vi "UpdatePrefKnown.vi"(0 "PrefItemNode in":refnum<k20>, 1 "UpdateResult":T1, 2 "error in (no error)":errorcluster) -> (3 "PrefItemNode out":refnum<k20>, 4 "Updated XML":string, 5 "Not Current":bool, 6 "error out":errorcluster)   [LabVIEW 2013, in "SetListPrefs.lvclass"]
uses:
  SetListPrefs.lvclass
  <resource>/objmgr/DOMUserDefRef.rc
  UpdateResult.ctl
  <vilib>/regexp/Match Regular Expression.xnode
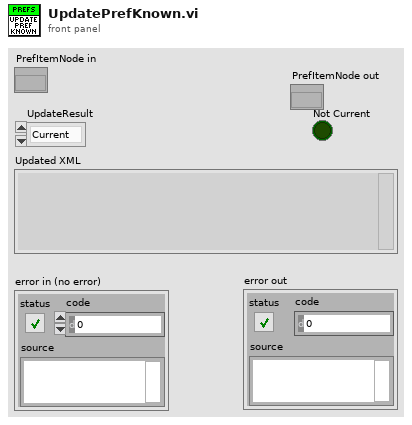
[diagram p1: front panel]
types:
  T1 = typedef "SetListPrefs.lvclass/UpdateResult.ctl" = enum16{"Current", "Old", "Unknown"}
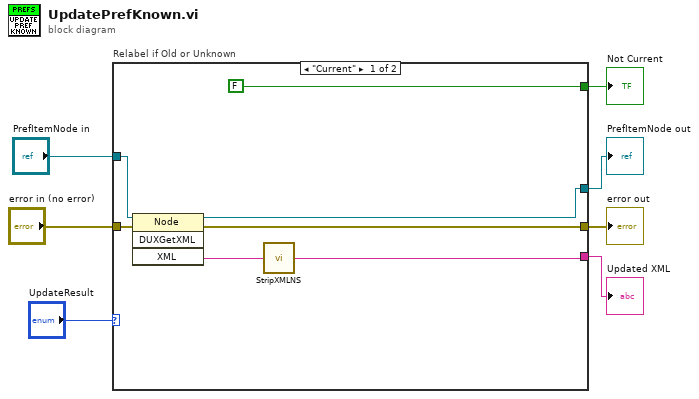
[diagram p0: block diagram]
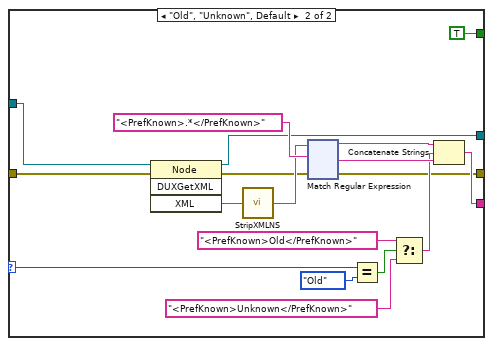
[diagram p2: hidden frame]
diagram:
  n1 = case "Relabel if Old or Unknown" shown="\"Current\"" "UpdateResult" {
    selector: "UpdateResult" -> [_ w28]
    tunnel: [w8 w29] -> w2
    tunnel: [FALSE TRUE] -> w1
    tunnel: "PrefItemNode in" -> [w11 w18]
    tunnel: "error in (no error)" -> [w12 w17]
    tunnel: [w10 w16] -> w4
    tunnel: [w13 w15] -> w3
    frame "Current" {
      n2 = invoke class="Node" method="DUXGetXML"(reference=w11, error in=w12) -> (reference out=w10:refnum<k20>, error out=w13:errorcluster, "XML"=w9:string)  [unwired: 2 in, 1 out]
      n3 = call "StripXMLNS.vi"("XML in"=w9) -> ("XML out"=w8:string)
    }
    frame "Old", "Unknown", Default {
      n4 = invoke class="Node" method="DUXGetXML"(reference=w18, error in=w17) -> (reference out=w16:refnum<k20>, error out=w19:errorcluster, "XML"=w20:string)  [unwired: 2 in, 1 out]
      n5 = call "StripXMLNS.vi"("XML in"=w20) -> ("XML out"=w21:string)
      n6 = xnode "Match Regular Expression"("input string"=w21, "regular expression"="<PrefKnown>.*</PrefKnown>", "error in"=w19) -> ("before match"=w31:string, "after match"=w30:string, "error out"=w15:errorcluster)  [unwired: 3 in, 2 out]
      n7 = Equal?(x=w28, y=UpdateResult."Old") -> (x = y?=w26:bool)
      n8 = Select(t="<PrefKnown>Old</PrefKnown>", s=w26, f="<PrefKnown>Unknown</PrefKnown>") -> (s? t:f=w25:string)
      n9 = Concatenate Strings(w31, w25, w30) -> (w29:string)
    }
  }
  "PrefItemNode out" <- w4
  "error out" <- w3
  "Updated XML" <- w2
  "Not Current" <- w1
